vi "Camera_Reconfig.vi"() -> ()   [LabVIEW 2022 SP3]
uses:
  <vilib>/vision/driver/IMAQdx.llb/IMAQdx Acquisition Mode.ctl
  <vilib>/vision/driver/NI_Vision_Acquisition_Software.lvlib
panel:
  out "Duration":u32
  in  "Stop":bool
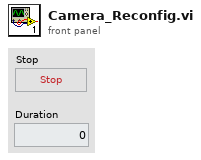
[diagram p1: front panel]
types:
  T1 = typedef "Data.ctl" = cluster{"system":cluster{"info":cluster{"menuSelect":u16, "version":u16, "serial":string, "captureActive":bool, "captureBegin":bool, "emptyAndRefill":bool}, "userInfo":cluster{"operatorName":string, "date":timestamp}, "camera":cluster{"exposureTime":i32, "aperture":enum32{"Item 0", "Item 1", "Item 2", "Item 3"}, "framerate":i32, "framerateMax":i32, "legacyAttributes":bool}}, "connections":cluster{"arduino":cluster{"connection":refnum<visa-resource-name>, "status":bool, "openState":bool, "emptyStart":u32}, "pump":cluster{"connection":refnum<visa-resource-name>, "status":bool, "command":string, "dispenseSpeed":i32, "flushSize":i32}, "camera":cluster{"cam1":cluster{"connection":T2, "status":bool}, "cam2":cluster{"connection":T2, "status":bool}}}, "queue":cluster{"process":cluster{"cam1":refnum<queue>, "cam2":refnum<queue>, "queueSize":i32}, "save":cluster{"cam1":refnum<queue>, "cam2":refnum<queue>, "queueSize":i32}, "overloadThreshold":i32}, "imageProcess":cluster{"cam1":cluster{"preAllocation":cluster{"image":T3, "originalDisplay":T3, "originalRgb":T3, "binary":T3, "save":T3, "calibrationFull":T3, "calibrationDetect":T3}, "calibration":cluster{"pathFull":path, "pathDetect":path, "ROI":T4}}, "cam2":cluster{"preAllocation":cluster{"image":T3, "originalDisplay":T3, "originalRgb":T3, "binary":T3, "save":T3, "calibrationFull":T3, "calibrationDetect":T3}, "calibration":cluster{"pathFull":path, "pathDetect":path, "ROI":T4}}, "process":cluster{"planeExtract":T3, "planeSubtract":T3, "cropMask":T3}, "detection":cluster{"sampleTimeout":i32, "sizeThreshold":i32, "detectionRegionPct":dbl}}, "sampleData":cluster{"sampleId":string, "projectId":string, "voucherID":string, "speciesName":string, "collectionDate":timestamp, "sampleStation":string, "location":string, "lat":dbl, "lon":dbl, "determiner":string, "sex":string, "otherNotes":string}, "Session In":T2}
  T2 = typedef "IMAQdx.ctl" = refnum<k21>
  T3 = typedef "IMAQ Image.ctl" = refnum<image>
  T4 = typedef "IMAQ Rectangle" = cluster{"Left":i32, "Top":i32, "Right":i32, "Bottom":i32, "Rotation":dbl}
  T5 = typedef "NI_Vision_Acquisition_Software.lvlib/IMAQdx Acquisition Mode.ctl" = enum32{"One Shot", "Continuous"}
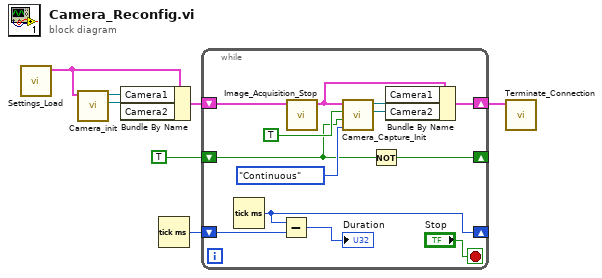
[diagram p0: block diagram]
diagram:
  n1 = call "Settings_Load.vi"() -> ("value"=w1:T1)  [unwired: 10 in, 1 out]
  n2 = call "Camera_init.vi"("input cluster"=w1) -> ("Camera2"=w6:T2, "Camera1"=w7:T2)  [unwired: 7 in, 2 out]
  n3 = Bundle By Name(cluster=w1, "Camera1"=w7, "Camera2"=w6) -> (w5:T1)
  n4 = Tick Count (ms)() -> (millisecond timer value=w3:u32)
  n5 = while {
    shift-right: [w14] -> w4
    shift-left: w5 -> [w15]
    shift-right: [w12] -> _
    shift-left: w3 -> [w11]
    shift-right: [w9] -> _
    shift-left: TRUE -> [w8]
    stop <- "Stop" stop-if-true
    n6 = Tick Count (ms)() -> (millisecond timer value=w12:u32)
    n7 = Subtract(x=w12, y=w11) -> (x-y=→"Duration":u32)
    n8 = call "Image_Acquisition_Stop.vi"("input cluster"=w15) -> ("output cluster"=w16:T1)  [unwired: 9 in, 1 out]
    n9 = call "Camera_Capture_Init.vi"("Continuous?"=IMAQdx_Acquisition_Mode."Continuous", "Detect Movement"=w8, "Crop?"=TRUE, "input cluster"=w16) -> ("Camera2"=w17:T2, "Camera1"=w18:T2)  [unwired: 6 in]
    n10 = Not(x=w8) -> (.not. x?=w9:bool)
    n11 = Bundle By Name(cluster=w16, "Camera1"=w18, "Camera2"=w17) -> (w14:T1)
  }
  n12 = call "Terminate_Connection.vi"("Data"=w4) -> ()  [unwired: 9 in, 2 out]
